vi "Handle Lap.vi"(8 "error in (no error)":errorcluster, 9 "Last Lap":dbl, 10 "Lap":u8, 11 "FormulaG App in":refnum<class "FormulaG App.lvclass">) -> (0 "error out":errorcluster, 2 "Finish":bool, 3 "FormulaG App out":refnum<class "FormulaG App.lvclass">, 5 "Fastest Lap":i32, 7 "Min Time":dbl)   [LabVIEW 2024, in "FormulaG.lvlib" / "FormulaG App.lvclass"]
uses:
  FormulaG App.lvclass
  FormulaG App.lvclass/FormulaG App.ctl
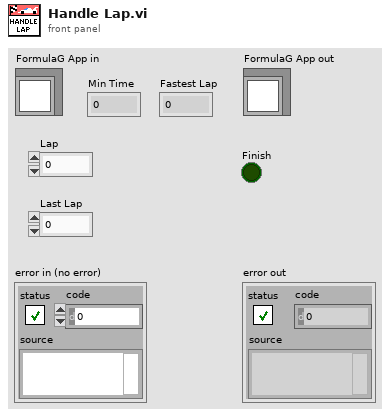
[diagram p1: front panel]
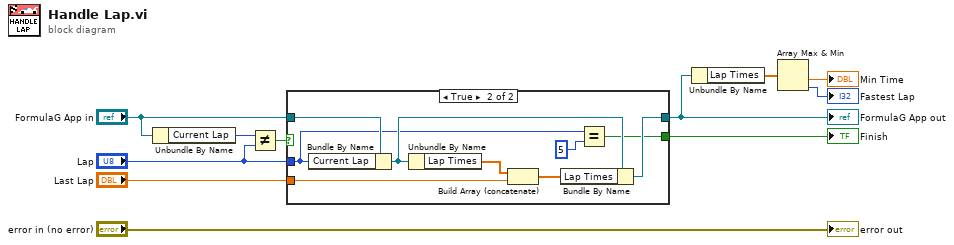
[diagram p0: block diagram]
diagram:
  n1 = Unbundle By Name("FormulaG App in") -> ("Current Lap"=w10:u8)
  n2 = Not Equal?(x=w10, y="Lap") -> (x != y?=w9:bool)
  n3 = case shown="True" w9 {
    tunnel: "Lap" -> [_ w15]
    tunnel: "Last Lap" -> [_ w19]
    tunnel: "FormulaG App in" -> [w12 w21]
    tunnel: [w12 w16] -> w1
    tunnel: [_ w13] -> w5
    frame False {
    }
    frame True {
      n4 = Bundle By Name(cluster=w21, "Current Lap"=w15) -> (w18:refnum<class "FormulaG App.lvclass">)
      n5 = Unbundle By Name(w18) -> ("Lap Times"=w20:dbl[])
      n6 = Build Array (concatenate)(w20, w19) -> (w17:dbl[])
      n7 = Bundle By Name(cluster=w18, "Lap Times"=w17) -> (w16:refnum<class "FormulaG App.lvclass">)
      n8 = Equal?(x=w15, y=u8 5) -> (x = y?=w13:bool)
    }
  }
  "FormulaG App out" <- w1
  "Finish" <- w5
  n9 = Unbundle By Name(w1) -> ("Lap Times"=w4:dbl[])
  n10 = Array Max & Min(array=w4) -> (min value=→"Min Time":dbl, min index (indices)=→"Fastest Lap":i32)  [unwired: 2 out]
  "error out" <- "error in (no error)"
